vi "ProdaNG.TestStepResult.Get.vi"(8 "error in (no error)":errorcluster, 9 "testStepId":i32, 10 "processStepResulttId":string, 11 "dbHandle":i32) -> (0 "error out":errorcluster, 1 "Found":bool, 2 "TestStepResult":T1, 3 "dbHandle out":i32)   [LabVIEW 2016]
doc: "This function returns a ProcessStepResult structure for a process result and a process step. \nParameter:\nhandle is an Integer, which is returned by the function Login() at the creation of a new connection.\nprocessResultId is the Id of the associated process result.\nprocessStepId is the Id of the associated process step.\nprocessStepResult is a pointer on a ProcessStepResult structure, which is filled if the returncode is 0. The structure must be defined in the calling program.\nReturncodes:\n0 No error\n< 0 ORACLE Error code\n6 (ERROR_INVALID_HANDLE) in case of an invalid handle\n1403 Record does not exist"
uses:
  Controls/ProdaNG.TestStepResult.ctl
  Controls/ProdaNG.TestStepResultSize.ctl
  prodllNG.dll
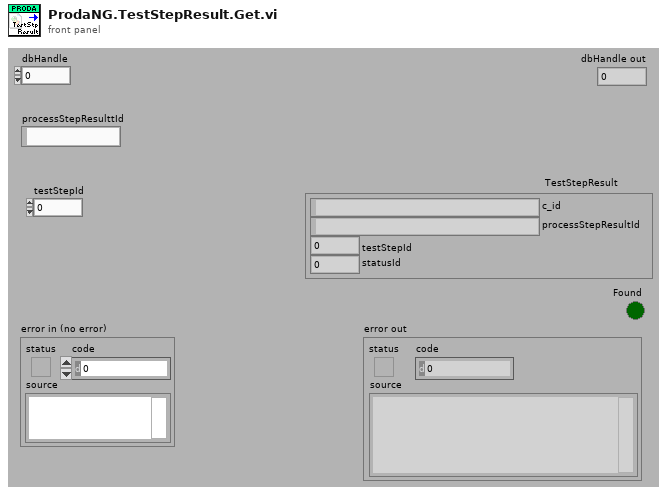
[diagram p1: front panel]
types:
  T1 = typedef "ProdaNG.TestStepResult.ctl" = cluster{"c_id":string, "processStepResultId":string, "testStepId":i32, "statusId":i32}
  T2 = typedef "ProdaNG.TestStepResultSize.ctl" = cluster{"c_id":i32, "processStepResultId":i32, "testStepId":i32, "statusId":i32}
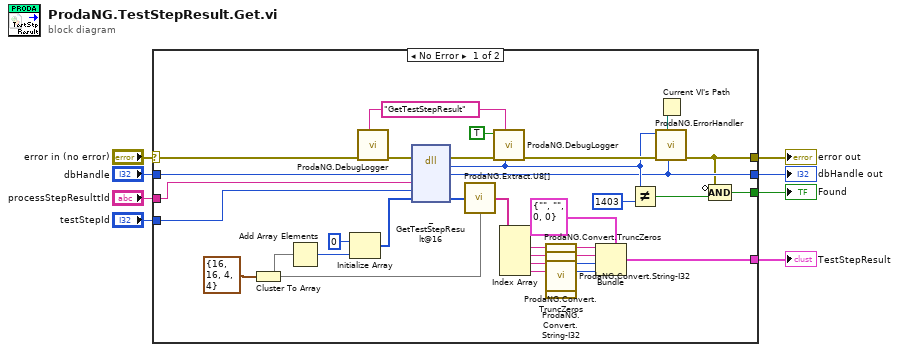
[diagram p0: block diagram]
diagram:
  n1 = case shown="No Error" "error in (no error)" {
    selector: "error in (no error)" -> [w19 w43]
    tunnel: [w10 w43] -> w7
    tunnel: "dbHandle" -> [w16 w42]
    tunnel: [w12 w42] -> w5
    tunnel: "processStepResulttId" -> [w17 _]
    tunnel: "testStepId" -> [w15 _]
    tunnel: [w14 _] -> w2
    tunnel: [w11 _] -> w1
    frame No Error {
      w40 = "GetTestStepResult" ("cmd")
      n2 = Cluster To Array(cluster=T2 {"c_id"=16, "processStepResultId"=16, "testStepId"=4, "statusId"=4} ("TestStepResultSize")) -> (array=w31:i32[])
      n3 = Add Array Elements(numeric array=w31) -> (sum=w34:i32)
      n4 = Initialize Array(u8 0 ("element"), w34) -> (w30:u8[])
      n5 = call "ProdaNG.DebugLogger.vi"("cmd"=w40, "error in (no error)"=w19) -> ("error out"=w38:errorcluster)  [unwired: 9 in]
      n6 = dll-call lib="D:/svn/LineTraceSystem/SOFTWARE/sources/Database/ProdaNG/prodllNG.dll" fn="_GetTestStepResult@16" ("ProDLL wrapper.dll:ProDLL_wrapper_GetWabcoParts_GetData")(error in=w38, "dbHandle"=w16, "processStepResultId"=w17, "testStepId"=w15, "testStepResult"=w30) -> (error out=w37:errorcluster, "return type"=w28:i32, "dbHandle"=w12:i32, "testStepResult"=w29:u8[])  [unwired: 4 in, 1 out]
      n7 = call "ProdaNG.Extract.U8[].vi"("unsigned byte array"=w29, "Sizes"=w31) -> ("Elements"=w33:string[])
      n8 = call "ProdaNG.DebugLogger.vi"("return type"=w28, "cmd"=w40, "error in (no error)"=w37, "done? (F)"=TRUE) -> ("error out"=w36:errorcluster)  [unwired: 7 in]
      n9 = Index Array(array=w33) -> (element #1=w21:string, element #2=w20:string, element #3=w27:string, element #4=w24:string)  [unwired: 4 in]
      n10 = call "ProdaNG.Convert.TruncZeros.vi"("string with \\0s"=w21) -> ("LV string"=w23:string)  [unwired: 10 in]
      n11 = call "ProdaNG.Convert.TruncZeros.vi"("string with \\0s"=w20) -> ("LV string"=w22:string)  [unwired: 10 in]
      n12 = call "ProdaNG.Convert.String-I32.vi"("unsigned byte string"=w27) -> ("32bit integer"=w26:i32)  [unwired: 10 in]
      n13 = call "ProdaNG.Convert.String-I32.vi"("unsigned byte string"=w24) -> ("32bit integer"=w25:i32)  [unwired: 10 in]
      n14 = Bundle(cluster=T1 {"c_id"="", "processStepResultId"="", "testStepId"=0, "statusId"=0} ("TestStepResult"), "c_id"=w23, "processStepResultId"=w22, "testStepId"=w26, "statusId"=w25) -> (w14:T1)
      n15 = Not Equal?(x=w28, y=1403) -> (x != y?=w13:bool)
      n16 = Current VI's Path() -> (path=w41:path)
      n17 = call "ProdaNG.ErrorHandler.vi"("dbHandleIn"=w12, "Path"=w41, "error in"=w36, "output_parameter"=w28) -> ("error out"=w10:errorcluster)  [unwired: 7 in]
      n18 = Compound Arithmetic op=AND(invert w10, w13) -> (w11:bool)
    }
    frame Error {
    }
  }
  "error out" <- w7
  "dbHandle out" <- w5
  "TestStepResult" <- w2
  "Found" <- w1
